vi "AFTInputFrame.vi"() -> ()   [LabVIEW 2012]
panel:
  in  "Model6Lo":dbl
  in  "Model5Lo":dbl
  in  "Model4Lo":dbl
  in  "Model3Lo":dbl
  in  "Model2Lo":dbl
  in  "Model1Lo":dbl
  out "Model6KparRange":string
  out "Model5KparRange":string
  out "Model4KparRange":string
  out "Model3KparRange":string
  out "Model2KparRange":string
  out "Model1KparRange":string
  in  "Model6Kpar":dbl
  in  "Model5Kpar":dbl
  in  "Model4Kpar":dbl
  in  "Model3Kpar":dbl
  in  "Model2Kpar":dbl
  in  "Model1Kpar":dbl
  in  "ModelPop6":bool caption="Population 6:"
  in  "ModelPop5":bool caption="Population 5:"
  in  "ModelPop4":bool caption="Population 4:"
  in  "ModelPop3":bool caption="Population 3:"
  in  "ModelPop2":bool caption="Population 2:"
  in  "ModelPop1":bool caption="Population 1:"
  in  "AgeDataGrid":i32(listbox)
  in  "NumD":dbl caption="NumD:"
  in  "RhoD":dbl caption="RhoD:"
  in  "AgeUncMode":string(combo) caption="Uncertainty mode:"
  in  "SigZeta":dbl caption="SigZeta:"
  in  "Zeta":dbl caption="Zeta:"
  in  "ZetaMode":string(combo) caption="Zeta mode:"
  in  "ImportAges":bool
  in  "LengthGOF":string(combo) caption="Goodness of fit method:"
  in  "ImportLengths":bool
  in  "LengthDataGrid":i32(listbox)
  in  "Populations":bool
  in  "Kpar1":string(combo) caption="Kinetic parameter:"
  in  "LengthReductionStdLabeled":dbl caption="Length reduction in standard:"
  in  "ConstantLo":dbl caption="µm"
  in  "DefaultLo":string(combo) caption="Default initial mean track length:"
  in  "UsedCf":bool caption="Used Cf Irradiation?"
  in  "ModelProjLength":bool caption="Model c-axis projected lengths?"
  in  "CAxisProj":string(combo) caption="C-axis projection:"
  in  "AnnealModel":string(combo) caption="Annealing model:"
  # "Model"
  # "Kpar range"
  # "Lo (µm):"
  # "Kpar"
  # "Length Data"
  # "Age Data"
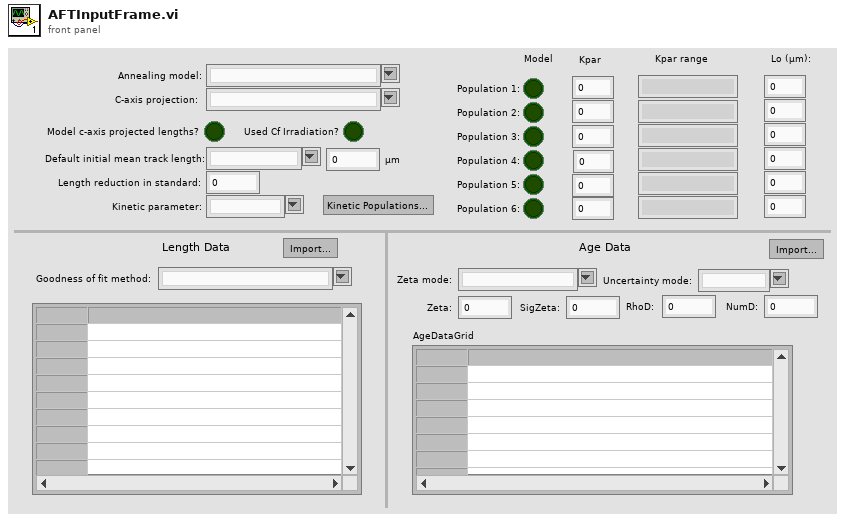
[diagram p1: front panel]
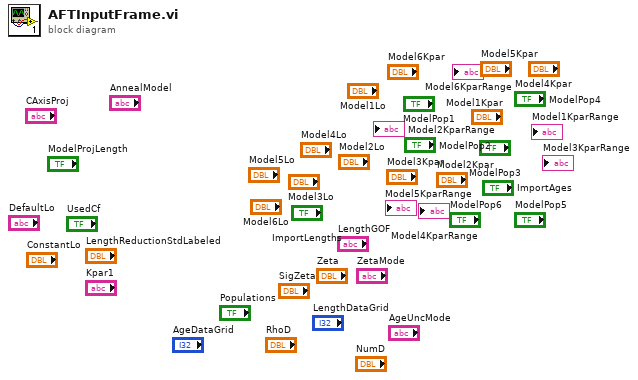
[diagram p0: block diagram]
diagram:
